vi "set edges settings.vi"(8 "error in (no error)":errorcluster, 10 "edges_settings":T1, 11 "id":i32) -> (0 "error out":errorcluster, 3 "function return":i32)   [LabVIEW 2012, in "libximc.lvlib"]
doc: "result_t XIMC_API set_edges_settings (device_t id, const edges_settings_t* edges_settings);"
uses:
  libximc.lvlib
  libximc.dll
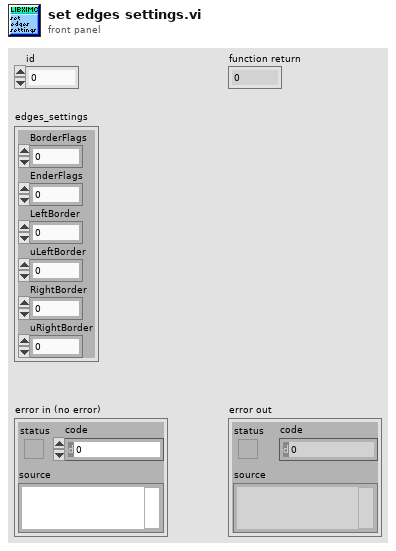
[diagram p1: front panel]
types:
  T1 = cluster{"BorderFlags":u32, "EnderFlags":u32, "LeftBorder":i32, "uLeftBorder":i32, "RightBorder":i32, "uRightBorder":i32}
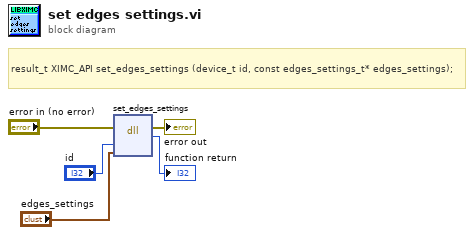
[diagram p0: block diagram]
diagram:
  # "result_t XIMC_API set_edges_settings (device_t id, const edges_settings_t* edges_settings);"
  n1 = dll-call lib="E:/labview-2.12.1-Labview_12.0/ximcLVx32/libximc.*" fn="set_edges_settings"(error in="error in (no error)", "id"="id", "edges_settings"="edges_settings") -> (error out=→"error out":errorcluster, →"function return":i32)  [unwired: 4 in, 1 out]
